vi "Get Object Parameter - JSON Tree.vi"(8 "error in (no error)":errorcluster, 10 "Parameter Name":string, 11 "JSON Tree In (JSON Object)":variant) -> (0 "error out":errorcluster, 1 "is JSON Null?":bool, 2 "JSON Value (JSON Tree)":variant, 3 "JSON Tree Out Passthrough":variant)   [LabVIEW 2011, in "i3-json.lvlib"]
doc: "Use this template to build a VI to use as a subVI."
uses:
  i3-json.lvlib
  JSON Types/JSON Type.ctl
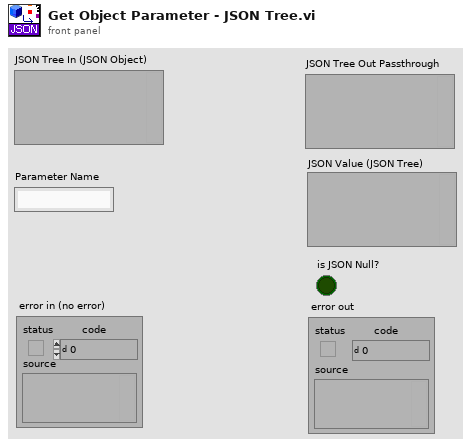
[diagram p1: front panel]
types:
  T1 = typedef "i3-json.lvlib/JSON Type.ctl" = enum8{"JSON Compatible", "JSON Array", "JSON Object", "JSON Null", "Double", "String", "Boolean", "Unknown", "Data JSON string"}
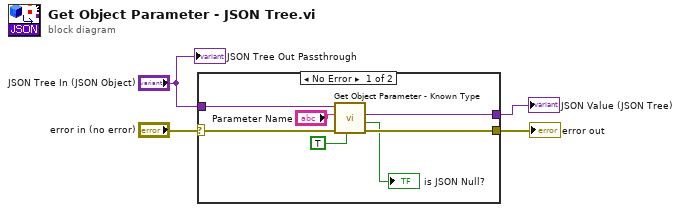
[diagram p0: block diagram]
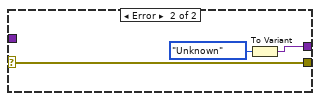
[diagram p2: hidden frame]
diagram:
  n1 = case shown="No Error" "error in (no error)" {
    selector: "error in (no error)" -> [w10 w14]
    tunnel: [w9 w14] -> w3
    tunnel: "JSON Tree In (JSON Object)" -> [w11 _]
    tunnel: [w8 w12] -> w2
    frame No Error {
      n2 = call "Get Object Parameter - Known Type.vi"("Get Value as JSON Tree? (F)"=TRUE, "error in (no error)"=w10, "Parameter Name"="Parameter Name", "JSON Tree In (JSON Object)"=w11) -> ("error out"=w9:errorcluster, "is JSON Null?"=→"is JSON Null?":bool, "Value"=w8:variant)  [unwired: 2 in, 3 out]
    }
    frame Error {
      n3 = To Variant(anything=JSON_Type."Unknown" ("JSON Type")) -> (Variant=w12:variant)
    }
  }
  "error out" <- w3
  "JSON Value (JSON Tree)" <- w2
  "JSON Tree Out Passthrough" <- "JSON Tree In (JSON Object)"
